vi "GetAllDeviceCommands.vi"(8 "error in":errorcluster, 11 "connection ID in":refnum<k5>) -> (0 "error out":errorcluster, 1 "Error Info":T1, 2 "Device Parameter Names":string[](array[string]), 3 "connection ID out":refnum<k5>, 4 "log string":string, 5 "OK":bool)   [LabVIEW 2020, in "ProdigyRemoteControl.lvlib"]
uses:
  ProdigyRemoteControl.lvlib
  DEFINITIONS/DEF_RcError.ctl
  DEFINITIONS/DEF_RcCmd.ctl
  <vilib>/regexp/Match Regular Expression.xnode
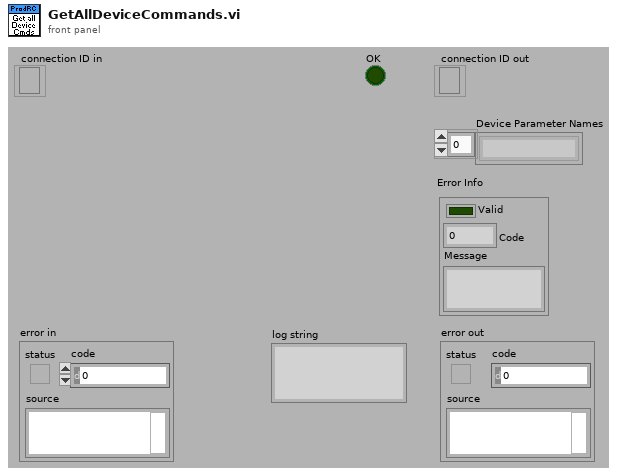
[diagram p1: front panel]
types:
  T1 = typedef "ProdigyRemoteControl.lvlib/DEF_RcError.ctl" = cluster{"Valid":bool, "Code":u16, "Message":string}
  T2 = typedef "ProdigyRemoteControl.lvlib/DEF_RcCmd.ctl" = string
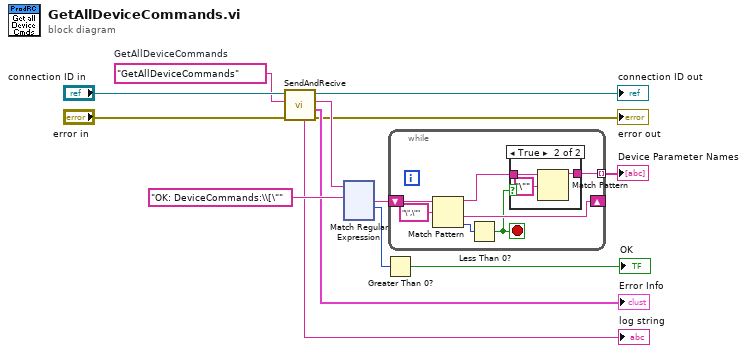
[diagram p0: block diagram]
diagram:
  w1 = T2 "GetAllDeviceCommands"  # GetAllDeviceCommands
  n1 = call "SendAndRecive.vi"("error in"="error in", "Command"=w1, "connection ID in"="connection ID in") -> ("error out"=→"error out":errorcluster, "Error Info"=→"Error Info":T1, "Answer"=w11:string, "connection ID out"=→"connection ID out":refnum<k5>, "Log String"=→"log string":string)  [unwired: 4 in]
  n2 = xnode "Match Regular Expression"("input string"=w11, "regular expression"="OK: DeviceCommands:\\[\"") -> ("after match"=w10:string, "offset past match"=w3:i32)  [unwired: 4 in, 3 out]
  n3 = Greater Than 0?(x=w3) -> (x > 0?=→"OK":bool)
  n4 = while {
    shift-right: [w17] -> _
    shift-left: w10 -> [w20]
    tunnel: [w15] -> w13 mode=indexing
    stop <- w14 stop-if-true
    n5 = Match Pattern(string=w20, regular expression="\",\"") -> (before substring=w16:string, after substring=w17:string, offset past match=w18:i32)  [unwired: 1 in, 1 out]
    n6 = Less Than 0?(x=w18) -> (x < 0?=w14:bool)
    n7 = case shown="True" w14 {
      tunnel: w16 -> [w21 w24]
      tunnel: [w21 w23] -> w15
      frame False {
      }
      frame True {
        n8 = Match Pattern(string=w24, regular expression="\"") -> (before substring=w23:string)  [unwired: 1 in, 3 out]
      }
    }
  }
  "Device Parameter Names" <- w13
